vi "svx_DAQ_CheckTriggerChannel.vi"(7 "State":T1={"Channel Info Array"=[], "Timing Mode"=enum."Time", "Timing Control 1"=25600.0, "Timing Control 2"=2560.0, "Timing Control 3"=16, "Timing Indicator 1"=0.1, "Reference Visible?"=FALSE, "Reference Type"=enum."<none>", "Tachometer Channel"="", "Tach Pulses Per Rev"=1, "Tach Direction"=enum."CW", "Tach Slope"=enum."Rising", "Tach Threshold"=0.0, "Trigger Channel"="", "Trigger Level"=20.0, "Pretrigger Samples"=1, "Trigger Slope"=enum."Falling", "Trigger Hysteresis"=0.0, "Logging Visible?"=FALSE, "Enable Logging"=FALSE, "Logfile Path"=path "c:/test.tdms"} {"Timing Control 2" format="%#_6f"; "Channel Info Array"."Max" min=0.0 format="± %^#_4g"; "Channel Info Array"."Channel Type" items=["Voltage (V)"=0, "Charge (C)"=9, "-"=99, "SPL (Pa)"=3, "Force (lbf)"=6, "Force (N)"=1, "Acceleration (g) - IEPE"=2, "Acceleration (g) - Charge"=12, "Acceleration (g) - 4 wire DC Voltage"=22, "Velocity (in/s)"=7, "Velocity (mm/s)"=8, "Prox Probe (mil)"=4, "Prox Probe (mm)"=5]}) -> (8 "Trigger Channel Invalid":bool)   [LabVIEW 2017, in "SVX NI-DAQmx AI Configuration XControl.xctl"]
uses:
  <vilib>/addons/Sound and Vibration/svt_DAQmx/Configuration XControl/SVX NI-DAQmx AI Configuration XControl.xctl
  <vilib>/addons/Sound and Vibration/svt_DAQmx/Configuration XControl/SubVIs/svx_DAQ_State.ctl
  <vilib>/addons/Sound and Vibration/svt_DAQmx/Configuration XControl/Controls/svx_DAQ_ChannelInfo.ctl
  <vilib>/addons/Sound and Vibration/svt_DAQmx/Configuration XControl/Controls/svx_DAQ_ChannelType.ctl
  <vilib>/addons/Sound and Vibration/svt_DAQmx/Configuration XControl/Controls/svx_DAQ_Coupling.ctl
  <vilib>/addons/Sound and Vibration/svt_DAQmx/Configuration XControl/Controls/svx_DAQ_Excitation.ctl
  <vilib>/addons/Sound and Vibration/svt_DAQmx/Configuration XControl/Controls/svx_DAQ_TimingType.ctl
  <vilib>/addons/Sound and Vibration/svt_DAQmx/Configuration XControl/Controls/svx_DAQ_ReferenceType.ctl
  <vilib>/addons/Sound and Vibration/svt_DAQmx/Configuration XControl/Controls/svx_DAQ_RotationDirection.ctl
  <vilib>/addons/Sound and Vibration/svt_DAQmx/Configuration XControl/Controls/svx_DAQ_Tach_Slope.ctl
  <vilib>/addons/Sound and Vibration/svt_DAQmx/Configuration XControl/Controls/svx_DAQ_Trigger_Slope.ctl
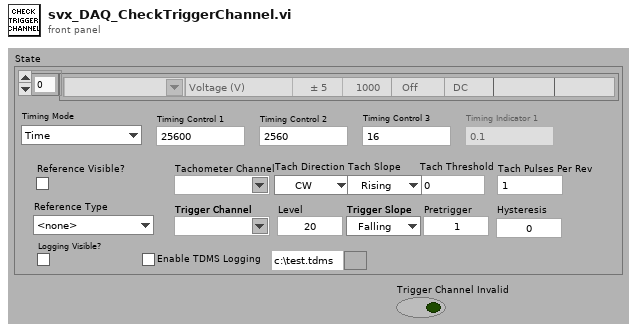
[diagram p1: front panel]
types:
  T1 = typedef "SVX NI-DAQmx AI Configuration XControl.xctl/svx_DAQ_State.ctl" = cluster{"Channel Info Array":T2[], "Timing Mode":T6, "Timing Control 1":dbl, "Timing Control 2":dbl, "Timing Control 3":i32, "Timing Indicator 1":dbl, "Reference Visible?":bool, "Reference Type":T7, "Tachometer Channel":string, "Tach Pulses Per Rev":i32, "Tach Direction":T8, "Tach Slope":T9, "Tach Threshold":dbl, "Trigger Channel":string, "Trigger Level":dbl, "Pretrigger Samples":i32, "Trigger Slope":T10, "Trigger Hysteresis":dbl, "Logging Visible?":bool, "Enable Logging":bool, "Logfile Path":path}
  T2 = typedef "SVX NI-DAQmx AI Configuration XControl.xctl/svx_DAQ_ChannelInfo.ctl" = cluster{"Initialized?":bool, "DAQmx Channel":tag, "Channel Type":T3, "Max":dbl, "Sensitivity":dbl, "Excitation":bool, "Coupling":T4, "Location":string, "Orientation":string, "excitation":T5}
  T3 = typedef "SVX NI-DAQmx AI Configuration XControl.xctl/svx_DAQ_ChannelType.ctl" = u16
  T4 = typedef "SVX NI-DAQmx AI Configuration XControl.xctl/svx_DAQ_Coupling.ctl" = enum16{"AC", "DC"}
  T5 = typedef "svx_DAQ_Excitation.ctl" = enum16{"Off", "Min", "Max"}
  T6 = typedef "SVX NI-DAQmx AI Configuration XControl.xctl/svx_DAQ_TimingType.ctl" = enum16{"Time", "Frequency", "Order"}
  T7 = typedef "SVX NI-DAQmx AI Configuration XControl.xctl/svx_DAQ_ReferenceType.ctl" = enum16{"<none>", "Analog Tachometer", "Analog SW Trigger"}
  T8 = typedef "SVX NI-DAQmx AI Configuration XControl.xctl/svx_DAQ_RotationDirection.ctl" = enum16{"CW", "CCW"}
  T9 = typedef "SVX NI-DAQmx AI Configuration XControl.xctl/svx_DAQ_Tach_Slope.ctl" = enum16{"Rising", "Falling"}
  T10 = typedef "SVX NI-DAQmx AI Configuration XControl.xctl/svx_DAQ_Trigger_Slope.ctl" = enum16{"Falling", "Rising"}
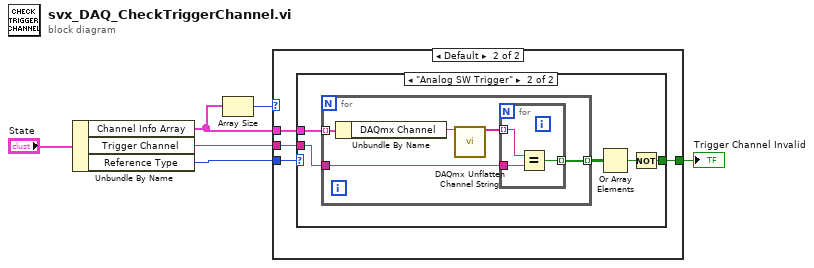
[diagram p0: block diagram]
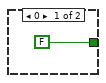
[diagram p2: hidden frame]
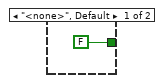
[diagram p3: hidden frame]
diagram:
  n1 = Unbundle By Name("State") -> ("Channel Info Array"=w3:T2[], "Trigger Channel"=w5:string, "Reference Type"=w1:T7)
  n2 = Array Size(array=w3) -> (size(s)=w2:i32)
  n3 = case shown="Default" w2 {
    tunnel: w5 -> [_ w11]
    tunnel: [FALSE w10] -> w4
    tunnel: w3 -> [_ w9]
    tunnel: w1 -> [_ w8]
    frame 0 {
    }
    frame Default {
      n4 = case shown="\"Analog SW Trigger\"" w8 {
        tunnel: w11 -> [_ w17]
        tunnel: [FALSE w14] -> w10
        tunnel: w9 -> [_ w13]
        frame "<none>", Default {
        }
        frame "Analog SW Trigger" {
          n5 = for {
            tunnel: w13 -> [w22] mode=indexing
            tunnel: w17 -> [w21]
            tunnel: [w20] -> w16 mode=indexing
            n6 = Unbundle By Name(w22) -> ("DAQmx Channel"=w19:tag)
            n7 = call <vilib>:"DAQmx Unflatten Channel String.vi"("names in"=w19) -> ("names out"=w18:string[])  [unwired: 13 in, 1 out]
            n8 = for {
              tunnel: w21 -> [w25]
              tunnel: [w24] -> w20 mode=indexing
              tunnel: w18 -> [w23] mode=indexing
              n9 = Equal?(x=w23, y=w25) -> (x = y?=w24:bool)
            }
          }
          n10 = Or Array Elements(Boolean array=w16) -> (logical OR=w15:bool)
          n11 = Not(x=w15) -> (.not. x?=w14:bool)
        }
      }
    }
  }
  "Trigger Channel Invalid" <- w4
